vi "Permute({b,c,h,w)_to_(bhw,c)).vi"(8 "error in":errorcluster, 11 "Features (bs, (c1+c2+...+cN), h, w)":sgl[][][][](array[numeric])) -> (0 "error out":errorcluster, 2 "Orig dims (bs, h, w, (c1+c2+...+cN))":i32[](array[numeric]), 3 "Features resshaped ((bs  x h x w),  c1+c1+..+ cN, )":sgl[][](array[numeric]), 5 "dT_Reshape":dbl format="%#_6p")   [LabVIEW 2020]
uses:
  <vilib>/Ngene/Deep Learning Toolkit/Toolkit/Deep_Learning_Toolkit_by_Ngene.lvlib
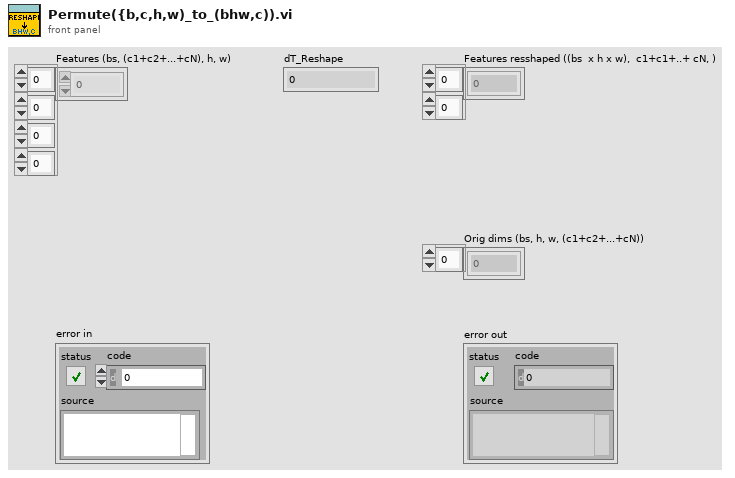
[diagram p1: front panel]
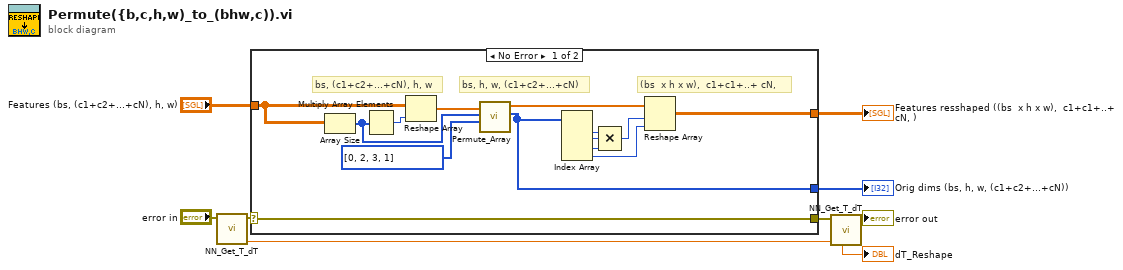
[diagram p0: block diagram]
diagram:
  n1 = call <vilib>:"NN_Get_T_dT.vi"("error in (no error)"="error in") -> ("T_out"=w2:dbl, "error out"=w3:errorcluster)  [unwired: 6 in, 1 out]
  n2 = case shown="No Error" w3 {
    selector: w3 -> [w10 w24]
    tunnel: [w23 _] -> w9
    tunnel: "Features (bs, (c1+c2+...+cN), h, w)" -> [w11 _]
    tunnel: [w22 _] -> w8
    tunnel: [w10 w24] -> w7
    frame No Error {
      # "(bs  x h x w),  c1+c1+..+ cN,"
      # "bs, h, w, (c1+c2+...+cN)"
      # "bs, (c1+c2+...+cN), h, w"
      n3 = Array Size(array=w11) -> (size(s)=w16:i32[])
      n4 = Multiply Array Elements(1:w16) -> (0:w12:i32)
      n5 = Reshape Array(w11, w12) -> (w13:sgl[])
      n6 = call "Permute_Array.vi"("permute_rule"=i32[] [0, 2, 3, 1] ("permute"), "Input_Dims"=w16, "1D Array In"=w13) -> ("Permuted_Dims"=w23:i32[], "1D Array out"=w15:sgl[])  [unwired: 7 in]
      n7 = Index Array(array=w23) -> (element #1=w18:i32, element #2=w19:i32, element #3=w20:i32, element #4=w17:i32)  [unwired: 4 in]
      n8 = Compound Arithmetic op=MULTIPLY(w18, w19, w20) -> (w21:i32)
      n9 = Reshape Array(w15, w21, w17) -> (w22:sgl[][])
    }
    frame Error {
    }
  }
  "Orig dims (bs, h, w, (c1+c2+...+cN))" <- w9
  "Features resshaped ((bs  x h x w),  c1+c1+..+ cN, )" <- w8
  n10 = call <vilib>:"NN_Get_T_dT.vi"("T_in"=w2, "error in (no error)"=w7) -> ("error out"=→"error out":errorcluster, "dT"=→"dT_Reshape":dbl)  [unwired: 5 in, 1 out]
